vi "Pad Calibration.vi"(8 "Error In":errorcluster, 11 "device ID":refnum<k1>) -> (0 "Error Out":errorcluster, 2 "Path to config file":path, 3 "device ID":refnum<k1>)   [LabVIEW 2014]
doc: "This VI calibrates game controller and saves settings into xml file"
uses:
  Controls/Controllers Clusters/Game Pad Calibration States.ctl
  Controls/Controllers Clusters/Game Pad Calibration Cluster.ctl
  <vilib>/Utility/xml.llb/Write to XML File(string).vi
  <vilib>/Utility/inputDevices.llb/joystickAcquire.vi
panel:
  in  "Summary Button":bool
  in  "Again Button":bool
  in  "Save Button":bool
  in  "button info":T1
  in  "axis info":T2
  in  "Finish Button":bool
  out "User Prompt":string caption="Final your calibration"
  # "Game Controller Calibration"
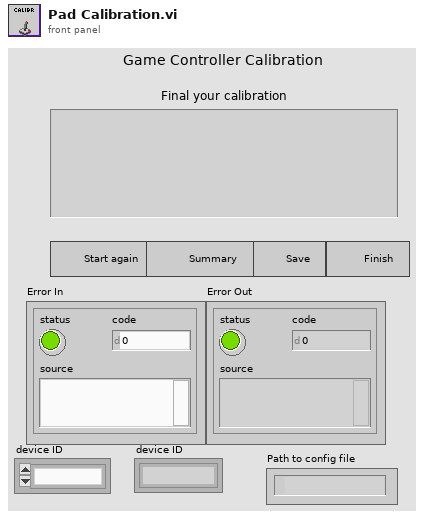
[diagram p1: front panel]
types:
  T1 = cluster{"button 1":bool, "button 2":bool, "button 3":bool, "button 4":bool, "button 5":bool, "button 6":bool, "button 7":bool, "button 8":bool, "button 9":bool, "button 10":bool, "button 11":bool, "button 12":bool, "button 13":bool, "button 14":bool, "button 15":bool, "button 16":bool, "button 17":bool, "button 18":bool, "button 19":bool, "button 20":bool, "button 21":bool, "button 22":bool, "button 23":bool, "button 24":bool, "button 25":bool, "button 26":bool, "button 27":bool, "button 28":bool, "button 29":bool, "button 30":bool, "button 31":bool, "button 32":bool}
  T2 = cluster{"X axis":i32, "Y axis":i32, "Z axis":i32, "X axis rotation":i32, "Y axis rotation":i32, "Z axis rotation":i32, "U axis":i32, "V axis":i32}
  T3 = typedef "Game Pad Calibration Cluster.ctl" = cluster{"Safety Button Number":u8, "Speed Axis Number":u8, "Speed Axis Max":i32, "Speed Axis Zero":i32, "Back Speed Axis Number":u8, "Back Speed Axis Max":i32, "Back Speed Axis Zero":i32, "Steering Axis Number":u8, "Steering Axis Max":i32, "Steering Axis Zero":i32}
  T4 = typedef "Game Pad Calibration States.ctl" = enum16{"Init", "Safety Button", "Speed Axis Max", "Speed Axis Zero", "Back Speed Axis Max", "Back Speed Axis Zero", "Right Axis Max", "Right Axis Zero", "Last Step", "Summary", "Save", "Exit"}
  T5 = enum8{"Enabled", "Disabled", "Disabled and Grayed Out"}
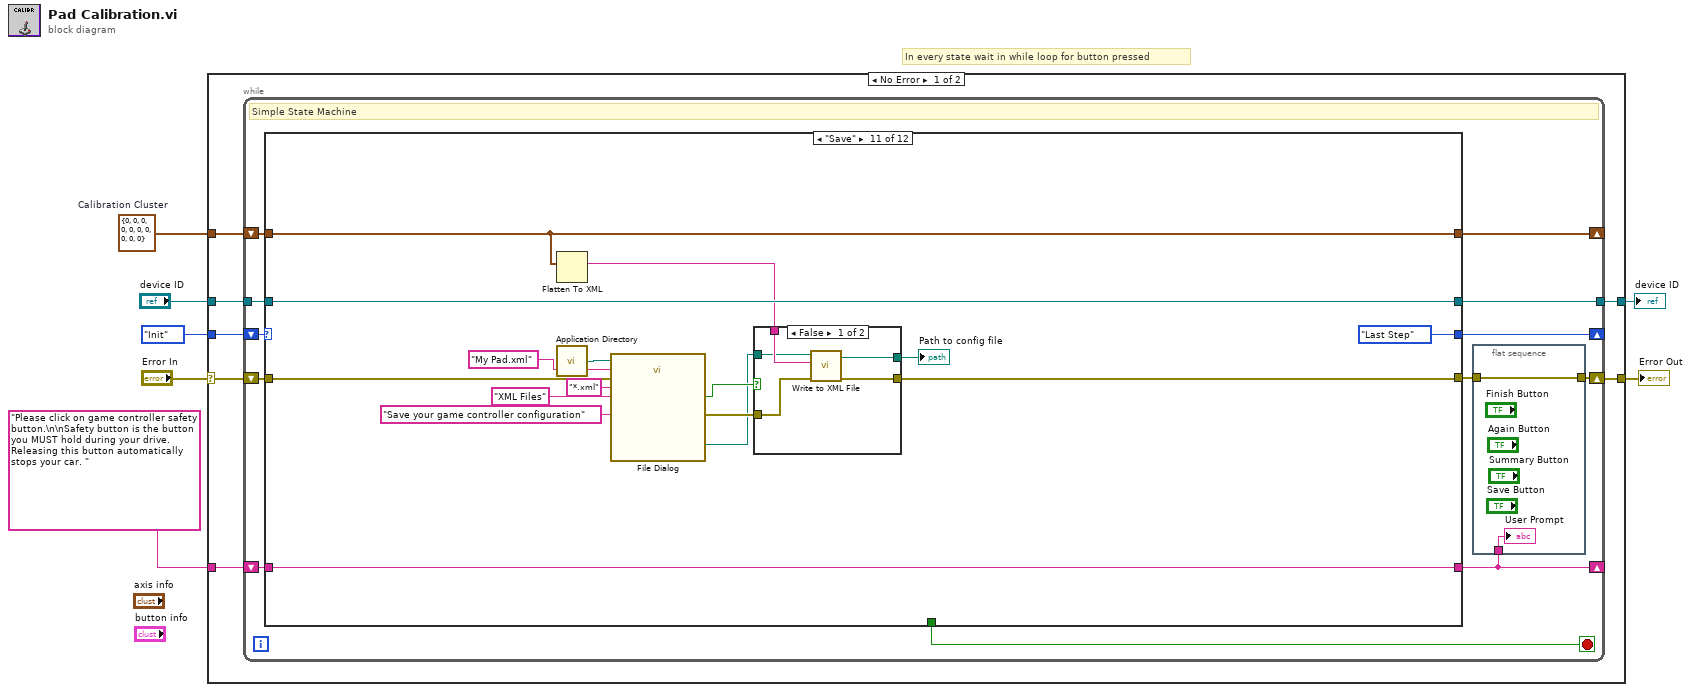
[diagram p0: block diagram]
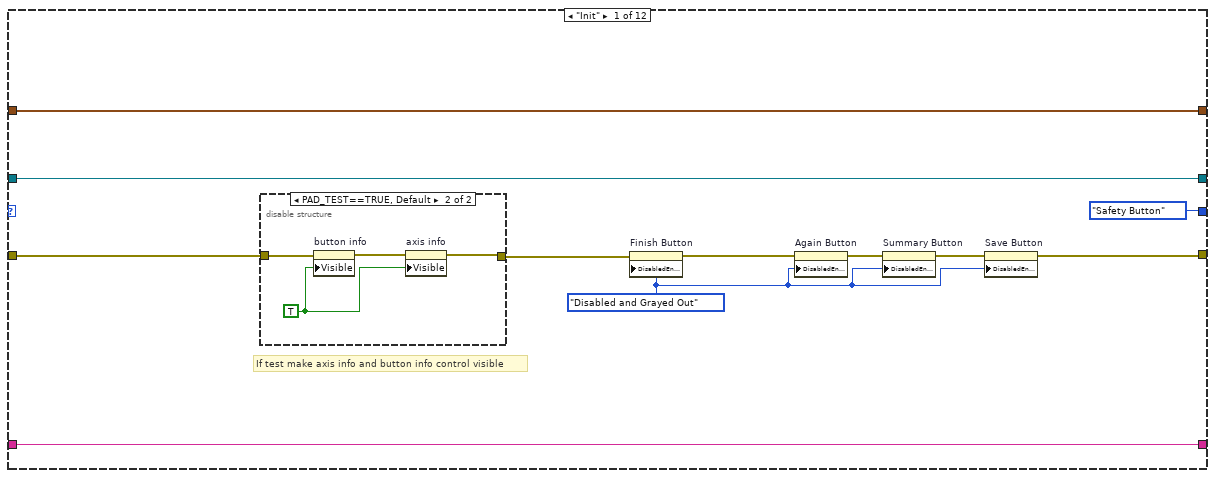
[diagram p2: hidden frame]
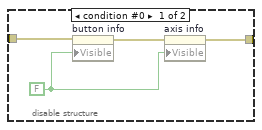
[diagram p3: hidden frame]
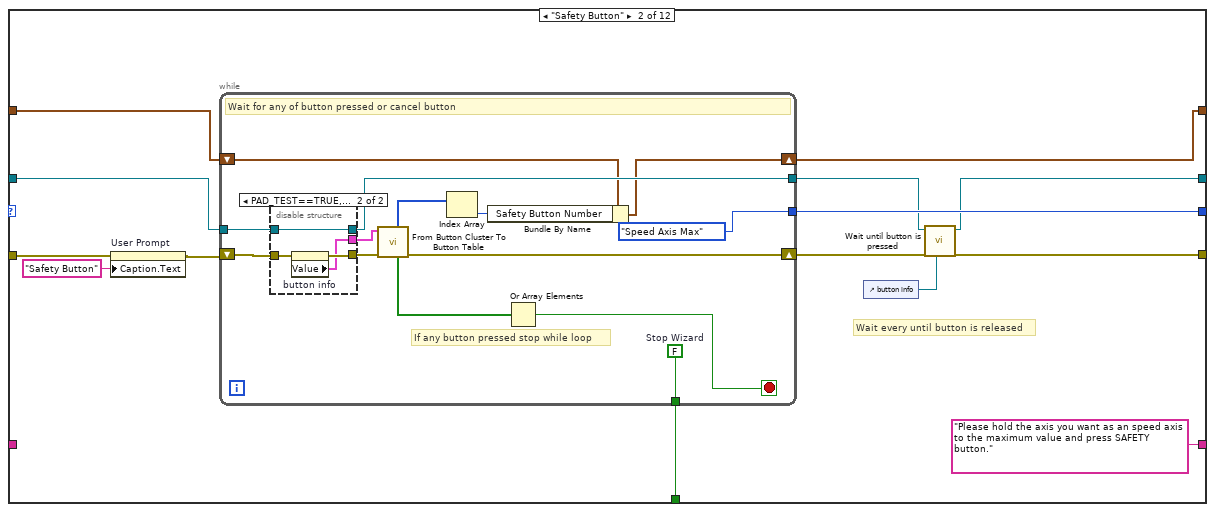
[diagram p4: hidden frame]
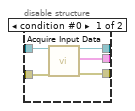
[diagram p5: hidden frame]
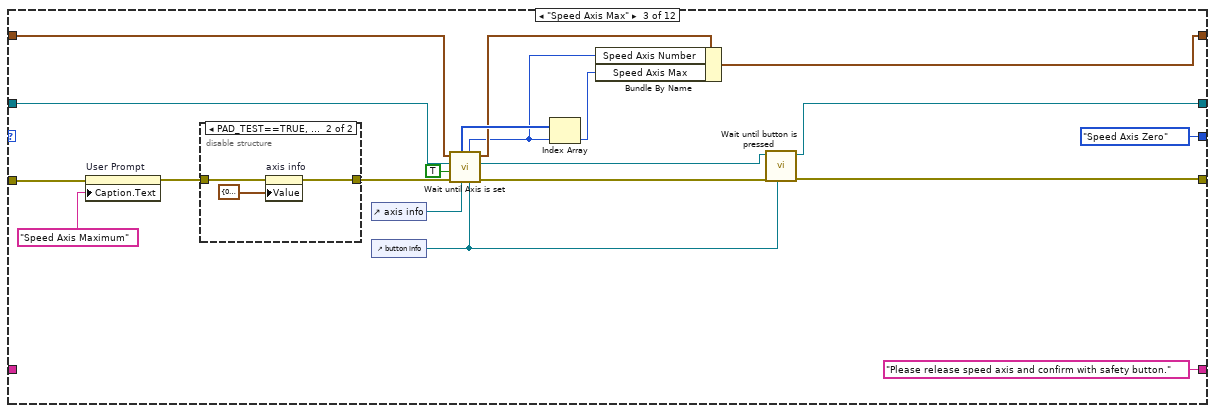
[diagram p6: hidden frame]
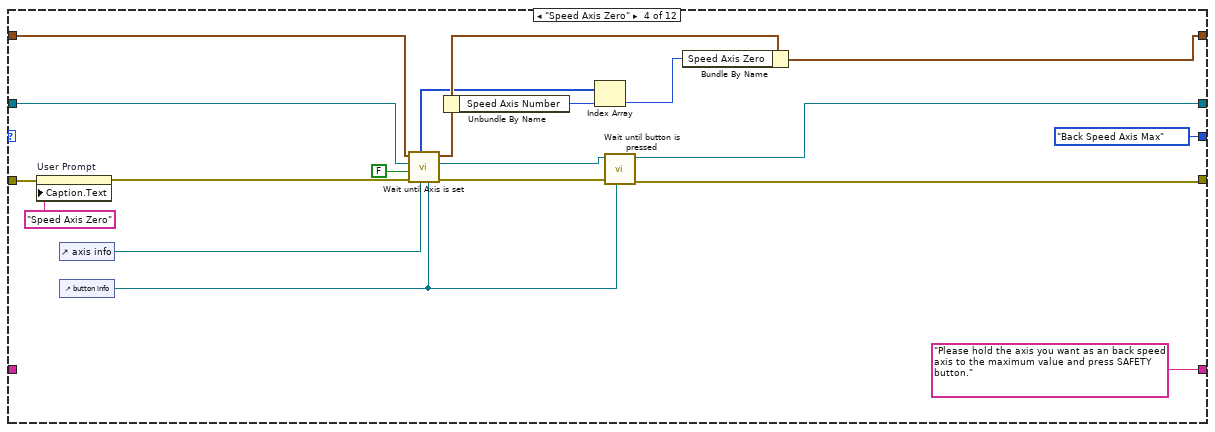
[diagram p8: hidden frame]
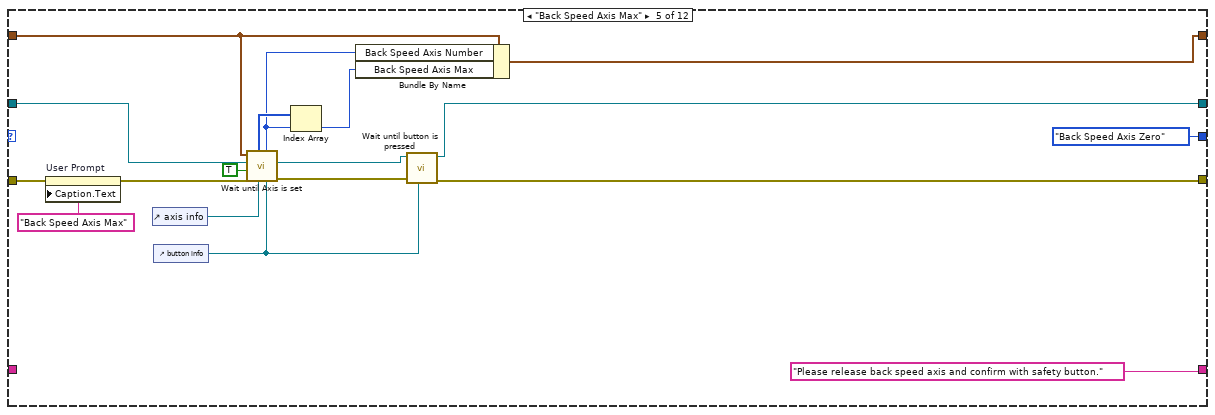
[diagram p9: hidden frame]
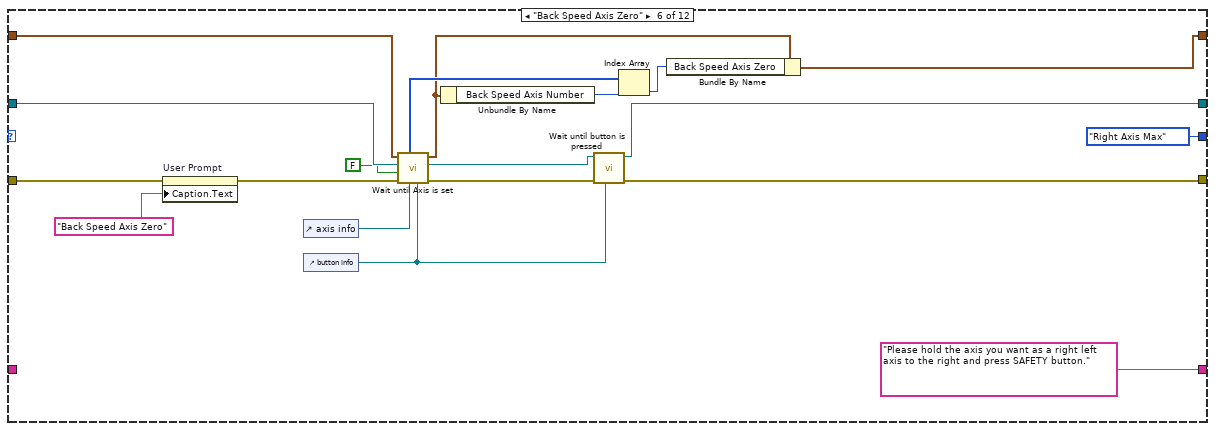
[diagram p10: hidden frame]
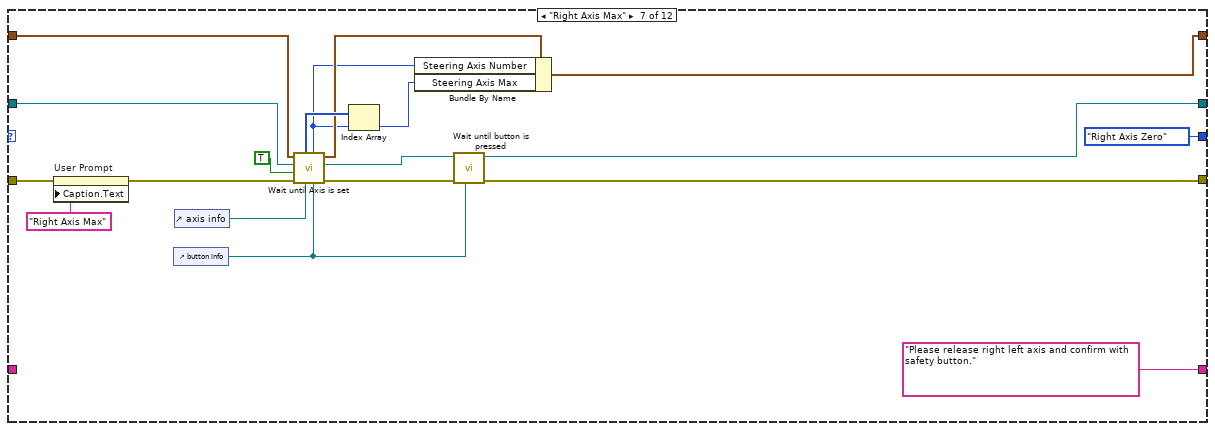
[diagram p11: hidden frame]
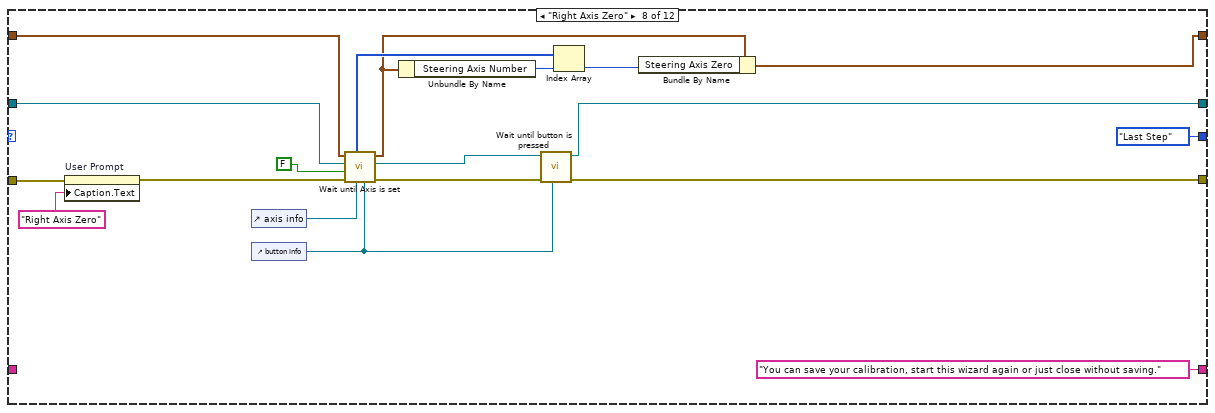
[diagram p12: hidden frame]
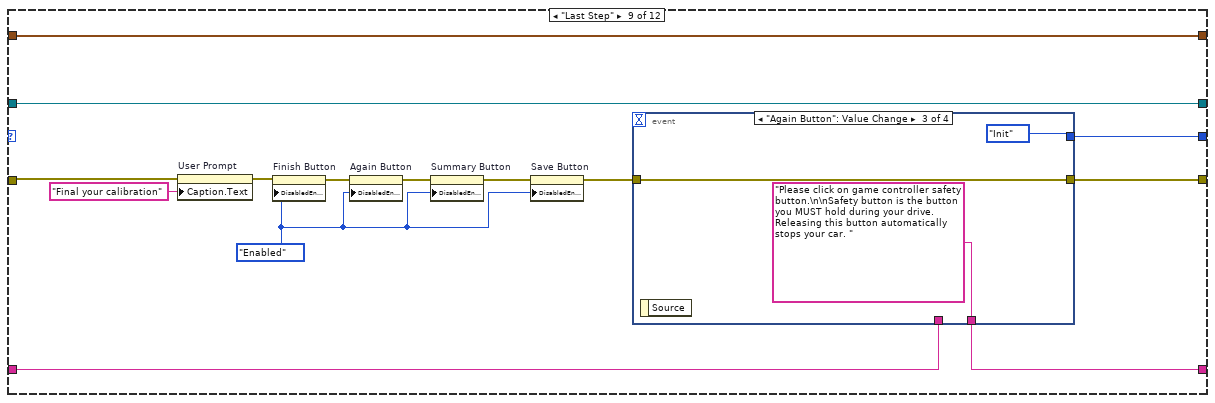
[diagram p13: hidden frame]
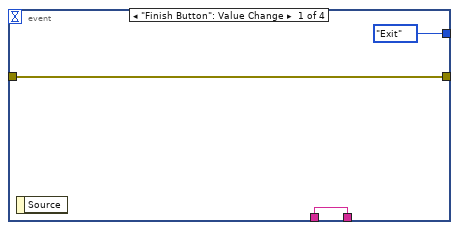
[diagram p14: hidden frame]
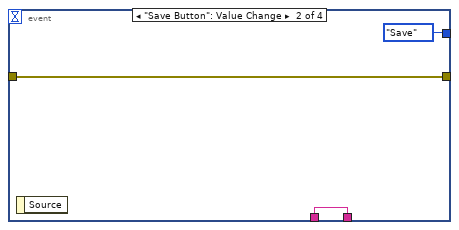
[diagram p15: hidden frame]
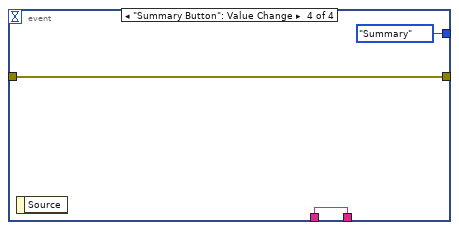
[diagram p16: hidden frame]
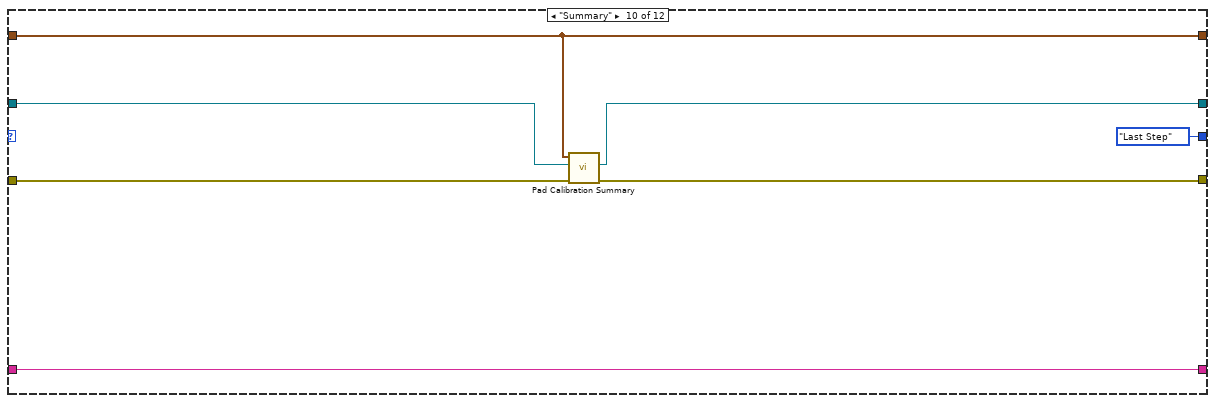
[diagram p17: hidden frame]
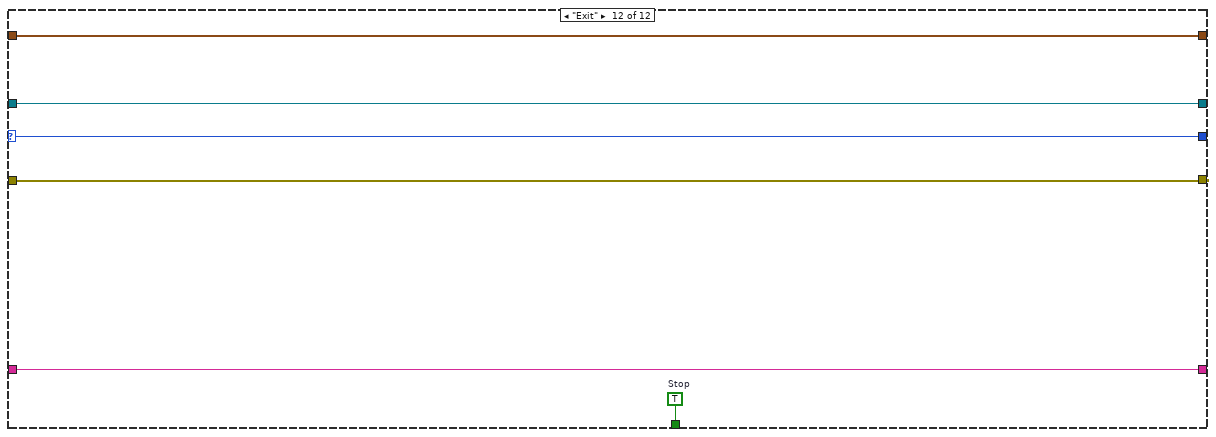
[diagram p19: hidden frame]
diagram:
  w2 = T3 {"Safety Button Number"=0, "Speed Axis Number"=0, "Speed Axis Max"=0, "Speed Axis Zero"=0, "Back Speed Axis Number"=0, "Back Speed Axis Max"=0, "Back Speed Axis Zero"=0, "Steering Axis Number"=0, "Steering Axis Max"=0, "Steering Axis Zero"=0}  # Calibration Cluster
  # "In every state wait in while loop for button pressed"
  n1 = case shown="No Error" "Error In" {
    selector: "Error In" -> [w14 w266]
    tunnel: [w12 w266] -> w6
    tunnel: Game_Pad_Calibration_States."Init" -> [w13 _]
    tunnel: "Please click on game controller safety button.\n\nSafety button is the button you MUST hold during your drive. Releasing this button automatically stops your car. " -> [w11 _]
    tunnel: "device ID" -> [w10 w265]
    tunnel: [w9 w265] -> w1
    tunnel: w2 -> [w8 _]
    frame No Error {
      n2 = while {
        shift-right: [w20] -> w12
        shift-left: w14 -> [w24]
        shift-right: [w25] -> _
        shift-left: w13 -> [w26]
        shift-right: [w19] -> _
        shift-left: w11 -> [w22]
        tunnel: w10 -> [w18]
        tunnel: [w17] -> w9
        shift-right: [w15] -> _
        shift-left: w8 -> [w16]
        stop <- w23 stop-if-true
        # "Simple State Machine"
        n3 = case shown="\"Save\"" w26 {
          selector: w26 -> [_ _ _ _ _ _ _ _ _ _ _ w264]
          tunnel: [Game_Pad_Calibration_States."Safety Button" w51 Game_Pad_Calibration_States."Speed Axis Zero" Game_Pad_Calibration_States."Back Speed Axis Max" Game_Pad_Calibration_States."Back Speed Axis Zero" Game_Pad_Calibration_States."Right Axis Max" Game_Pad_Calibration_States."Right Axis Zero" Game_Pad_Calibration_States."Last Step" w209 Game_Pad_Calibration_States."Last Step" Game_Pad_Calibration_States."Last Step" w264] -> w25
          tunnel: [w30 w52 w89 w113 w135 w163 w183 w197 w208 w232 w247 w263] -> w21
          tunnel: w24 -> [w36 w60 w104 w126 w144 w149 w173 w201 w204 w233 w242 w263]
          tunnel: [_ w59 _ _ _ _ _ _ _ _ _ w262] -> w23
          tunnel: w22 -> [w38 _ _ _ _ _ _ _ w206 w234 w250 w261]
          tunnel: [w38 "Please hold the axis you want as an speed axis to the maximum value and press SAFETY button." "Please release speed axis and confirm with safety button." "Please hold the axis you want as an back speed axis to the maximum value and press SAFETY button." "Please release back speed axis and confirm with safety button." "Please hold the axis you want as a right left axis to the right and press SAFETY button." "Please release right left axis and confirm with safety button." "You can save your calibration, start this wizard again or just close without saving." w207 w234 w250 w261] -> w19
          tunnel: w18 -> [w34 w56 w101 w121 w139 w161 w174 w192 w216 w230 w249 w259]
          tunnel: [w34 w48 w87 w112 w138 w158 w176 w190 w216 w229 w249 w259] -> w17
          tunnel: w16 -> [w37 w55 w100 w122 w134 w162 w179 w191 w215 w231 w248 w260]
          tunnel: [w37 w58 w92 w119 w133 w153 w168 w186 w215 w231 w248 w260] -> w15
          frame "Init" {
            w29 = T5."Disabled and Grayed Out" ("Disabled")
            # "If test make axis info and button info control visible"
            n4 = disable-structure shown="PAD_TEST==TRUE, Default" {
              disable-tunnel: w36 -> [w43 w47]
              disable-tunnel: [w41 w45] -> w35
              frame condition #0 {
                w40 = FALSE
                n5 = property on="button info" class="Clust (strict)"(error in=w43, "Visible"=w40) -> (error out=w42:errorcluster)  [unwired: 1 in, 1 out]
                n6 = property on="axis info" class="Clust (strict)"(error in=w42, "Visible"=w40) -> (error out=w41:errorcluster)  [unwired: 1 in, 1 out]
              }
              frame condition #1 (active) {
                w44 = TRUE
                n7 = property on="button info" class="Clust (strict)"(error in=w47, "Visible"=w44) -> (error out=w46:errorcluster)  [unwired: 1 in, 1 out]
                n8 = property on="axis info" class="Clust (strict)"(error in=w46, "Visible"=w44) -> (error out=w45:errorcluster)  [unwired: 1 in, 1 out]
              }
            }
            n9 = property on="Finish Button" class="Bool"(error in=w35, "DisabledEnum"=w29) -> (error out=w33:errorcluster)  [unwired: 1 in, 1 out]
            n10 = property on="Again Button" class="Bool"(error in=w33, "DisabledEnum"=w29) -> (error out=w32:errorcluster)  [unwired: 1 in, 1 out]
            n11 = property on="Summary Button" class="Bool"(error in=w32, "DisabledEnum"=w29) -> (error out=w31:errorcluster)  [unwired: 1 in, 1 out]
            n12 = property on="Save Button" class="Bool"(error in=w31, "DisabledEnum"=w29) -> (error out=w30:errorcluster)  [unwired: 1 in, 1 out]
          }
          frame "Safety Button" {
            # "Wait every until button is released"
            n13 = property on="User Prompt" class="Str"(error in=w60, "Caption.Text"="Safety Button") -> (error out=w54:errorcluster)  [unwired: 1 in, 1 out]
            n14 = while {
              shift-right: [w72] -> w53
              shift-left: w54 -> [w73]
              tunnel: [w74] -> w59
              tunnel: [Game_Pad_Calibration_States."Speed Axis Max"] -> w51
              tunnel: w56 -> [w70]
              tunnel: [w69] -> w49
              shift-right: [w67] -> w58
              shift-left: w55 -> [w68]
              stop <- w75 stop-if-true
              w74 = FALSE  # Stop Wizard
              # "If any button pressed stop while loop"
              # "Wait for any of button pressed or cancel button"
              n15 = disable-structure shown="PAD_TEST==TRUE, Default" {
                disable-tunnel: w73 -> [w80 w83]
                disable-tunnel: w70 -> [w79 w84]
                disable-tunnel: [w78 w84] -> w69
                disable-tunnel: [w77 w81] -> w66
                disable-tunnel: [w76 w82] -> w65
                frame condition #0 {
                  n16 = call-poly <vilib>:"Acquire Input Data.vi"("device ID"=w79, "error in (no error)"=w80) -> ("device ID"=w78:refnum<k1>, "button info"=w77:T1, "error out"=w76:errorcluster)  [unwired: 13 in, 2 out]
                }
                frame condition #1 (active) {
                  n17 = property on="button info" class="Clust (strict)"(error in=w83) -> (error out=w82:errorcluster, "Value"=w81:T1)  [unwired: 1 in, 1 out]
                }
              }
              n18 = call "From Button Cluster To Button Table.vi"("Error In"=w65, "button info"=w66) -> ("Error Out"=w72:errorcluster, "Buttons array"=w64:bool[], "Which ones?"=w63:u8[])  [unwired: 7 in]
              n19 = Index Array(array=w63) -> (element=w62:u8)  [unwired: 1 in]
              n20 = Bundle By Name(cluster=w68, "Safety Button Number"=w62) -> (w67:T3)
              n21 = Or Array Elements(Boolean array=w64) -> (logical OR=w75:bool)
            }
            n22 = control-ref of="button info"() -> (w50:refnum<vi>)
            n23 = call "Wait until button is pressed.vi"("Button Info"=w50, "error in (no error)"=w53, "device ID in"=w49) -> ("error out"=w52:errorcluster, "Device ID out"=w48:refnum<k1>)  [unwired: 7 in]
          }
          frame "Speed Axis Max" {
            n24 = property on="User Prompt" class="Str"(error in=w104, "Caption.Text"="Speed Axis Maximum") -> (error out=w97:errorcluster)  [unwired: 1 in, 1 out]
            n25 = disable-structure shown="PAD_TEST==TRUE, Default" {
              disable-tunnel: w97 -> [w105 w108]
              disable-tunnel: [w105 w107] -> w96
              frame condition #0 {
              }
              frame condition #1 (active) {
                n26 = property on="axis info" class="Clust (strict)"(error in=w108, "Value"=T2 {"X axis"=0, "Y axis"=0, "Z axis"=0, "X axis rotation"=0, "Y axis rotation"=0, "Z axis rotation"=0, "U axis"=0, "V axis"=0} ("axis info")) -> (error out=w107:errorcluster)  [unwired: 1 in, 1 out]
              }
            }
            n27 = control-ref of="axis info"() -> (w99:refnum<vi>)
            n28 = control-ref of="button info"() -> (w86:refnum<vi>)
            n29 = call "Wait until Axis is set.vi"("Button Info"=w86, "Axis Info"=w99, "error in (no error)"=w96, "Maximum?"=TRUE, "device ID in"=w101, "Calibration Cluster in"=w100) -> ("error out"=w90:errorcluster, "Device ID out"=w88:refnum<k1>, "Calibration Cluster out"=w95:T3, "index"=w94:i32, "Axis Array"=w98:i32[])  [unwired: 1 in]
            n30 = Index Array(array=w98, index=w94) -> (element=w93:i32)
            n31 = Bundle By Name(cluster=w95, "Speed Axis Number"=w94, "Speed Axis Max"=w93) -> (w92:T3)
            n32 = call "Wait until button is pressed.vi"("Button Info"=w86, "error in (no error)"=w90, "device ID in"=w88) -> ("error out"=w89:errorcluster, "Device ID out"=w87:refnum<k1>)  [unwired: 7 in]
          }
          frame "Speed Axis Zero" {
            n33 = property on="User Prompt" class="Str"(error in=w126, "Caption.Text"="Speed Axis Zero") -> (error out=w124:errorcluster)  [unwired: 1 in, 1 out]
            n34 = control-ref of="axis info"() -> (w120:refnum<vi>)
            n35 = control-ref of="button info"() -> (w110:refnum<vi>)
            n36 = call "Wait until Axis is set.vi"("Button Info"=w110, "Axis Info"=w120, "error in (no error)"=w124, "Maximum?"=FALSE, "device ID in"=w121, "Calibration Cluster in"=w122) -> ("error out"=w114:errorcluster, "Device ID out"=w111:refnum<k1>, "Calibration Cluster out"=w118:T3, "Axis Array"=w117:i32[])  [unwired: 1 in, 1 out]
            n37 = Unbundle By Name(w118) -> ("Speed Axis Number"=w116:u8)
            n38 = Index Array(array=w117, index=w116) -> (element=w115:i32)
            n39 = call "Wait until button is pressed.vi"("Button Info"=w110, "error in (no error)"=w114, "device ID in"=w111) -> ("error out"=w113:errorcluster, "Device ID out"=w112:refnum<k1>)  [unwired: 7 in]
            n40 = Bundle By Name(cluster=w118, "Speed Axis Zero"=w115) -> (w119:T3)
          }
          frame "Back Speed Axis Max" {
            n41 = property on="User Prompt" class="Str"(error in=w144, "Caption.Text"="Back Speed Axis Max") -> (error out=w142:errorcluster)  [unwired: 1 in, 1 out]
            n42 = control-ref of="axis info"() -> (w136:refnum<vi>)
            n43 = control-ref of="button info"() -> (w129:refnum<vi>)
            n44 = call "Wait until Axis is set.vi"("Button Info"=w129, "Axis Info"=w136, "error in (no error)"=w142, "Maximum?"=TRUE, "device ID in"=w139, "Calibration Cluster in"=w134) -> ("error out"=w141:errorcluster, "Device ID out"=w140:refnum<k1>, "index"=w131:i32, "Axis Array"=w132:i32[])  [unwired: 1 in, 1 out]
            n45 = Index Array(array=w132, index=w131) -> (element=w130:i32)
            n46 = Bundle By Name(cluster=w134, "Back Speed Axis Number"=w131, "Back Speed Axis Max"=w130) -> (w133:T3)
            n47 = call "Wait until button is pressed.vi"("Button Info"=w129, "error in (no error)"=w141, "device ID in"=w140) -> ("error out"=w135:errorcluster, "Device ID out"=w138:refnum<k1>)  [unwired: 7 in]
          }
          frame "Back Speed Axis Zero" {
            n48 = property on="User Prompt" class="Str"(error in=w149, "Caption.Text"="Back Speed Axis Zero") -> (error out=w148:errorcluster)  [unwired: 1 in, 1 out]
            n49 = control-ref of="axis info"() -> (w156:refnum<vi>)
            n50 = control-ref of="button info"() -> (w157:refnum<vi>)
            n51 = call "Wait until Axis is set.vi"("Button Info"=w157, "Axis Info"=w156, "error in (no error)"=w148, "Maximum?"=FALSE, "device ID in"=w161, "Calibration Cluster in"=w162) -> ("error out"=w164:errorcluster, "Device ID out"=w159:refnum<k1>, "Calibration Cluster out"=w154:T3, "Axis Array"=w155:i32[])  [unwired: 1 in, 1 out]
            n52 = Unbundle By Name(w154) -> ("Back Speed Axis Number"=w152:u8)
            n53 = call "Wait until button is pressed.vi"("Button Info"=w157, "error in (no error)"=w164, "device ID in"=w159) -> ("error out"=w163:errorcluster, "Device ID out"=w158:refnum<k1>)  [unwired: 7 in]
            n54 = Index Array(array=w155, index=w152) -> (element=w151:i32)
            n55 = Bundle By Name(cluster=w154, "Back Speed Axis Zero"=w151) -> (w153:T3)
          }
          frame "Right Axis Max" {
            n56 = property on="User Prompt" class="Str"(error in=w173, "Caption.Text"="Right Axis Max") -> (error out=w171:errorcluster)  [unwired: 1 in, 1 out]
            n57 = control-ref of="button info"() -> (w177:refnum<vi>)
            n58 = control-ref of="axis info"() -> (w178:refnum<vi>)
            n59 = call "Wait until Axis is set.vi"("Button Info"=w177, "Axis Info"=w178, "error in (no error)"=w171, "Maximum?"=TRUE, "device ID in"=w174, "Calibration Cluster in"=w179) -> ("error out"=w182:errorcluster, "Device ID out"=w181:refnum<k1>, "Calibration Cluster out"=w169:T3, "index"=w167:i32, "Axis Array"=w170:i32[])  [unwired: 1 in]
            n60 = Index Array(array=w170, index=w167) -> (element=w166:i32)
            n61 = Bundle By Name(cluster=w169, "Steering Axis Number"=w167, "Steering Axis Max"=w166) -> (w168:T3)
            n62 = call "Wait until button is pressed.vi"("Button Info"=w177, "error in (no error)"=w182, "device ID in"=w181) -> ("error out"=w183:errorcluster, "Device ID out"=w176:refnum<k1>)  [unwired: 7 in]
          }
          frame "Right Axis Zero" {
            n63 = property on="User Prompt" class="Str"(error in=w201, "Caption.Text"="Right Axis Zero") -> (error out=w199:errorcluster)  [unwired: 1 in, 1 out]
            n64 = control-ref of="axis info"() -> (w195:refnum<vi>)
            n65 = control-ref of="button info"() -> (w194:refnum<vi>)
            n66 = call "Wait until Axis is set.vi"("Button Info"=w194, "Axis Info"=w195, "error in (no error)"=w199, "Maximum?"=FALSE, "device ID in"=w192, "Calibration Cluster in"=w191) -> ("error out"=w198:errorcluster, "Device ID out"=w193:refnum<k1>, "Calibration Cluster out"=w187:T3, "Axis Array"=w188:i32[])  [unwired: 1 in, 1 out]
            n67 = Unbundle By Name(w187) -> ("Steering Axis Number"=w189:u8)
            n68 = call "Wait until button is pressed.vi"("Button Info"=w194, "error in (no error)"=w198, "device ID in"=w193) -> ("error out"=w197:errorcluster, "Device ID out"=w190:refnum<k1>)  [unwired: 7 in]
            n69 = Index Array(array=w188, index=w189) -> (element=w185:i32)
            n70 = Bundle By Name(cluster=w187, "Steering Axis Zero"=w185) -> (w186:T3)
          }
          frame "Last Step" {
            w210 = T5."Enabled" ("Disabled")
            n71 = property on="User Prompt" class="Str"(error in=w204, "Caption.Text"="Final your calibration") -> (error out=w205:errorcluster)  [unwired: 1 in, 1 out]
            n72 = property on="Finish Button" class="Bool"(error in=w205, "DisabledEnum"=w210) -> (error out=w214:errorcluster)  [unwired: 1 in, 1 out]
            n73 = property on="Again Button" class="Bool"(error in=w214, "DisabledEnum"=w210) -> (error out=w213:errorcluster)  [unwired: 1 in, 1 out]
            n74 = property on="Summary Button" class="Bool"(error in=w213, "DisabledEnum"=w210) -> (error out=w212:errorcluster)  [unwired: 1 in, 1 out]
            n75 = property on="Save Button" class="Bool"(error in=w212, "DisabledEnum"=w210) -> (error out=w211:errorcluster)  [unwired: 1 in, 1 out]
            n76 = event shown="[2] \"Again Button\": Value Change" {
              selector: _ -> [_ _ _ _]
              dyn-events: _ -> [_ _ _ _]
              timeout: _ -> [_ _ _ _]
              tunnel: w211 -> [w218 w221 w224 w227]
              tunnel: [Game_Pad_Calibration_States."Exit" Game_Pad_Calibration_States."Save" Game_Pad_Calibration_States."Init" Game_Pad_Calibration_States."Summary"] -> w209
              tunnel: [w218 w221 w224 w227] -> w208
              tunnel: [w217 w220 "Please click on game controller safety button.\n\nSafety button is the button you MUST hold during your drive. Releasing this button automatically stops your car. " w226] -> w207
              tunnel: w206 -> [w217 w220 _ w226]
              event "Finish Button": Value Change {
                n77 = event-data() -> ()  [unwired: 1 in, 1 out]
              }
              event "Save Button": Value Change {
                n78 = event-data() -> ()  [unwired: 1 in, 1 out]
              }
              event "Again Button": Value Change {
                n79 = event-data() -> ()  [unwired: 1 in, 1 out]
              }
              event "Summary Button": Value Change {
                n80 = event-data() -> ()  [unwired: 1 in, 1 out]
              }
            }
          }
          frame "Summary" {
            n81 = call "Pad Calibration Summary.vi"("Error In"=w233, "device ID"=w230, "Calibration Cluster"=w231) -> ("Error Out"=w232:errorcluster, "device ID out"=w229:refnum<k1>)  [unwired: 7 in]
          }
          frame "Save" {
            n82 = Flatten To XML(anything=w248) -> (xml string=w246:string)
            n83 = call <vilib>:"Application Directory.vi"() -> ("Application Directory"=w245:path)
            n84 = call "File Dialog"("start path"=w245, "prompt"="Save your game controller configuration", "default name"="My Pad.xml", "error in"=w242, "pattern (all files)"="*.xml", "pattern label"="XML Files") -> ("selected path"=w237:path, "cancelled"=w238:bool, "error out"=w243:errorcluster)  [unwired: 6 in, 1 out]
            n85 = case shown="False" w238 {
              tunnel: [w256 w258] -> w247
              tunnel: w246 -> [w255 _]
              tunnel: w243 -> [w254 w258]
              tunnel: w237 -> [w253 w257]
              tunnel: [w252 w257] -> w236
              frame False {
                n86 = call-poly <vilib>:"Write to XML File.vi"("error in (no error)"=w254, "XML Input"=w255, "XML File Path"=w253) -> ("error out"=w256:errorcluster, "XML File Path(duplicate)"=w252:path)  [unwired: 6 in, 1 out]
              }
              frame True {
              }
            }
            "Path to config file" <- w236
          }
          frame "Exit" {
            w262 = TRUE  # Stop
          }
        }
        n87 = flat-sequence {
          tunnel: w21 -> [w28]
          tunnel: [w28] -> w20
          tunnel: w19 -> [w27]
          frame #0 {
            "User Prompt" <- w27
          }
        }
      }
    }
    frame Error {
    }
  }
  "Error Out" <- w6
  "device ID" <- w1
